vi "tt20panel_DO_lifetime.vi"(8 "error in (no error)":errorcluster, 9 "corr_settings":T1, 10 "stop_counts":refnum<queue>, 11 "tt20panel in":refnum<class "tt20panel.lvclass">) -> (0 "error out":errorcluster, 3 "tt20panel out":refnum<class "tt20panel.lvclass">)   [LabVIEW 2015, in "tt20panel.lvclass"]
uses:
  tt20panel.lvclass
  tt20_class/tt20_histo_settings_tdef.ctl
  tt20_class/tt20.lvclass
  UI/panel_class/panel.lvclass
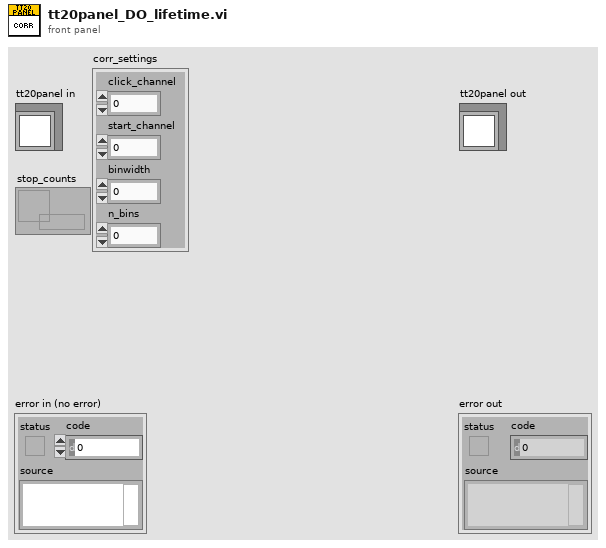
[diagram p1: front panel]
types:
  T1 = typedef "tt20_histo_settings_tdef.ctl" = cluster{"click_channel":u32, "start_channel":u32, "binwidth":i64, "n_bins":i32}
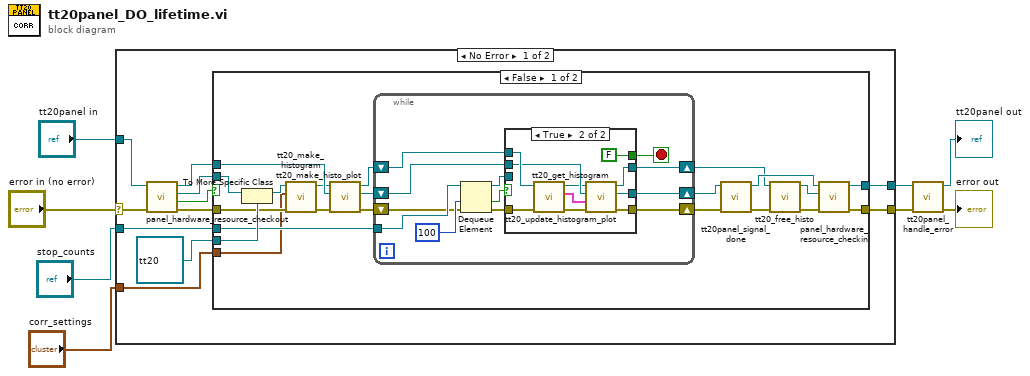
[diagram p0: block diagram]
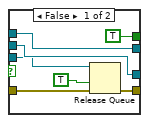
[diagram p2: hidden frame]
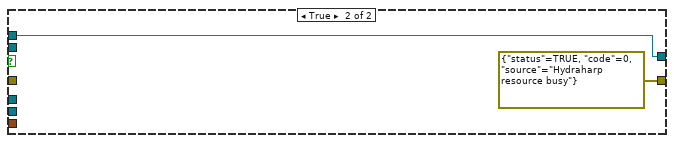
[diagram p3: hidden frame]
diagram:
  n1 = case shown="No Error" "error in (no error)" {
    selector: "error in (no error)" -> [w18 w73]
    tunnel: [w15 w73] -> w6
    tunnel: [w12 w72] -> w2
    tunnel: "tt20panel in" -> [w19 w72]
    tunnel: "stop_counts" -> [w10 _]
    tunnel: "corr_settings" -> [w9 _]
    frame No Error {
      n2 = call "panel_hardware_resource_checkout.vi"("error in (no error)"=w18, "panel in"=w19) -> ("error out"=w16:errorcluster, "timed out?"=w17:bool, "hardware.lvclass"=w13:refnum<class "hardware.lvclass">, "panel out"=w14:refnum<class "tt20panel.lvclass">)  [unwired: 6 in]
      n3 = case shown="False" w17 {
        tunnel: w16 -> [w32 _]
        tunnel: [w38 errorcluster {"status"=TRUE, "code"=0, "source"="Hydraharp resource busy"} ("error out")] -> w15
        tunnel: w14 -> [w27 w70]
        tunnel: w13 -> [w39 _]
        tunnel: refnum<class "tt20.lvclass"> refnum ("tt20.lvclass") -> [w40 _]
        tunnel: [w37 w70] -> w12
        tunnel: w10 -> [w36 _]
        tunnel: w9 -> [w24 _]
        frame False {
          n4 = To More Specific Class(target class=w40, reference=w39) -> (specific class reference=w31:refnum<class "tt20.lvclass">)  [unwired: 1 in, 1 out]
          n5 = call "tt20_make_histogram.vi"("error in (no error)"=w32, "histo_settings"=w24, "tt20 in"=w31) -> ("error out"=w30:errorcluster, "tt20 out"=w26:refnum<class "tt20.lvclass">)  [unwired: 7 in]
          n6 = call "tt20_make_histo_plot.vi"("error in (no error)"=w30, "panel in"=w27, "tt20 in"=w26) -> ("error out"=w29:errorcluster, "panel out"=w28:refnum<class "tt20panel.lvclass">, "tt20 out"=w25:refnum<class "tt20.lvclass">)  [unwired: 6 in]
          n7 = while {
            tunnel: w36 -> [w52]
            shift-right: [w44] -> w35
            shift-left: w29 -> [w50]
            shift-right: [w45] -> w22
            shift-left: w25 -> [w47]
            shift-right: [w43] -> w34
            shift-left: w28 -> [w46]
            stop <- w42 stop-if-true
            n8 = Dequeue Element(queue=w52, timeout in ms (-1)=100, error in (no error)=w50) -> (queue out=w41:refnum<queue>, timed out?=w49:bool, error out=w48:errorcluster)  [unwired: 1 out]
            n9 = case shown="True" w49 {
              tunnel: w48 -> [w55 w67]
              tunnel: w47 -> [w58 w68]
              tunnel: w46 -> [w57 w66]
              tunnel: [w58 w64] -> w45
              tunnel: [w54 w61] -> w44
              tunnel: [w57 w65] -> w43
              tunnel: [TRUE FALSE] -> w42
              tunnel: w41 -> [w56 _]
              frame False {
                n10 = Release Queue(queue=w56, force destroy? (F)=TRUE, error in (no error)=w55) -> (error out=w54:errorcluster)  [unwired: 2 out]
              }
              frame True {
                n11 = call "tt20_get_histogram.vi"("error in (no error)"=w67, "tt20 in"=w68) -> ("error out"=w62:errorcluster, "histogram"=w60:cluster{dbl[], dbl[]}[], "tt20 out"=w63:refnum<class "tt20.lvclass">)  [unwired: 7 in]
                n12 = call "tt20_update_histogram_plot.vi"("error in (no error)"=w62, "histogram"=w60, "tt20panel in"=w66, "tt20 in"=w63) -> ("error out"=w61:errorcluster, "panel out"=w65:refnum<class "tt20panel.lvclass">, "tt20 out"=w64:refnum<class "tt20.lvclass">)  [unwired: 5 in]
              }
            }
          }
          n13 = call "tt20panel_signal_done.vi"("error in (no error)"=w35, "tt20panel in"=w34) -> ("error out"=w23:errorcluster, "tt20panel out"=w33:refnum<class "tt20panel.lvclass">)  [unwired: 8 in]
          n14 = call "tt20_free_histo.vi"("error in (no error)"=w23, "tt20 in"=w22) -> ("error out"=w20:errorcluster, "tt20 out"=w21:refnum<class "tt20.lvclass">)  [unwired: 8 in]
          n15 = call "panel_hardware_resource_checkin.vi"("error in (no error)"=w20, "hardware.lvclass"=w21, "panel in"=w33) -> ("error out"=w38:errorcluster, "panel out"=w37:refnum<class "tt20panel.lvclass">)  [unwired: 7 in]
        }
        frame True {
        }
      }
    }
    frame Error {
    }
  }
  n16 = call "tt20panel_handle_error.vi"("error in (no error)"=w6, "tt20panel in"=w2) -> ("error out"=→"error out":errorcluster, "tt20panel out"=→"tt20panel out":refnum<class "tt20panel.lvclass">)  [unwired: 8 in]
